vi "CmdExe.Split Output Data to StdOut, StdError, and Return Code.vi"(8 "error in":errorcluster, 11 "Output Data":string) -> (0 "error out":errorcluster, 1 "Return Code":i32, 2 "StdError":string, 3 "StdOut":string)   [LabVIEW 2018]
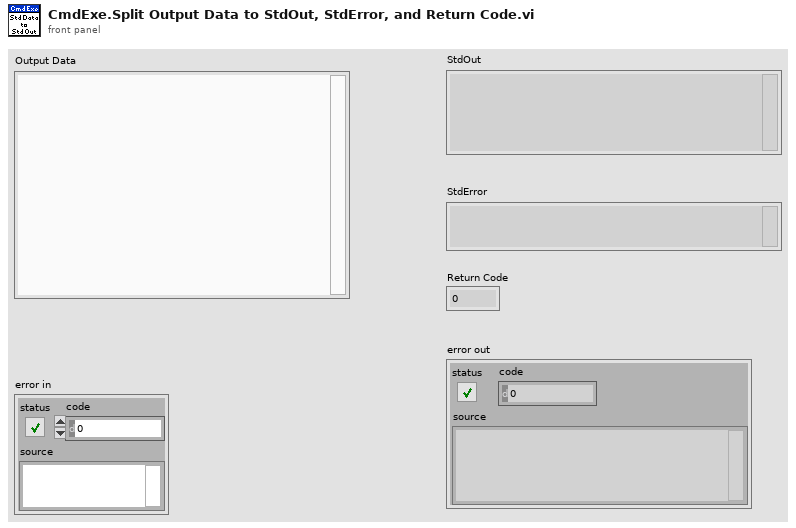
[diagram p1: front panel]
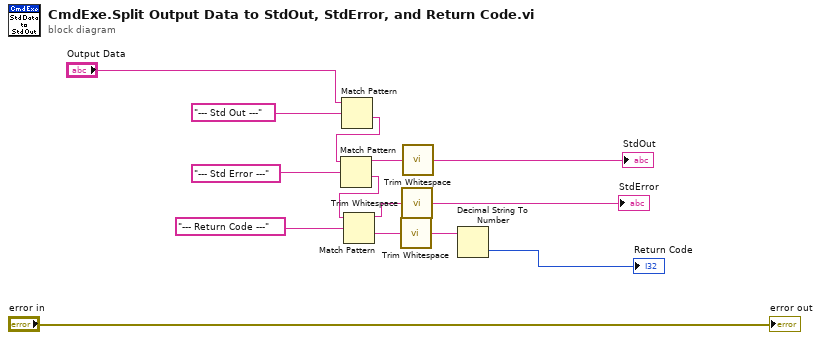
[diagram p0: block diagram]
diagram:
  n1 = Match Pattern(string="Output Data", regular expression="--- Std Out ---") -> (after substring=w7:string)  [unwired: 1 in, 3 out]
  n2 = Match Pattern(string=w7, regular expression="--- Std Error ---") -> (before substring=w6:string, after substring=w8:string)  [unwired: 1 in, 2 out]
  n3 = Match Pattern(string=w8, regular expression="--- Return Code ---") -> (before substring=w9:string, after substring=w10:string)  [unwired: 1 in, 2 out]
  n4 = call <vilib>:"Trim Whitespace.vi"("string"=w10) -> ("trimmed string"=w5:string)  [unwired: 1 in]
  n5 = call <vilib>:"Trim Whitespace.vi"("string"=w9) -> ("trimmed string"=→"StdError":string)  [unwired: 1 in]
  n6 = call <vilib>:"Trim Whitespace.vi"("string"=w6) -> ("trimmed string"=→"StdOut":string)  [unwired: 1 in]
  n7 = Decimal String To Number(string=w5) -> (number=→"Return Code":i32)  [unwired: 2 in, 1 out]
  "error out" <- "error in"
